vi "StartCapture.vi"(0 "object in":refnum<class "Hamamatsu.lvclass">, 5 "error in (no error)":errorcluster) -> (14 "object out":refnum<class "Hamamatsu.lvclass">, 19 "error out":errorcluster)   [LabVIEW 2019, in "Hamamatsu.lvclass"]
uses:
  Hamamatsu.lvclass
  Hamamatsu.lvclass/Hamamatsu.ctl
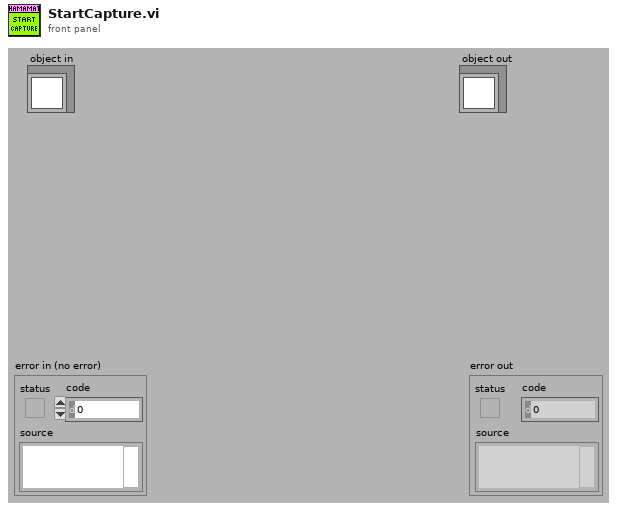
[diagram p1: front panel]
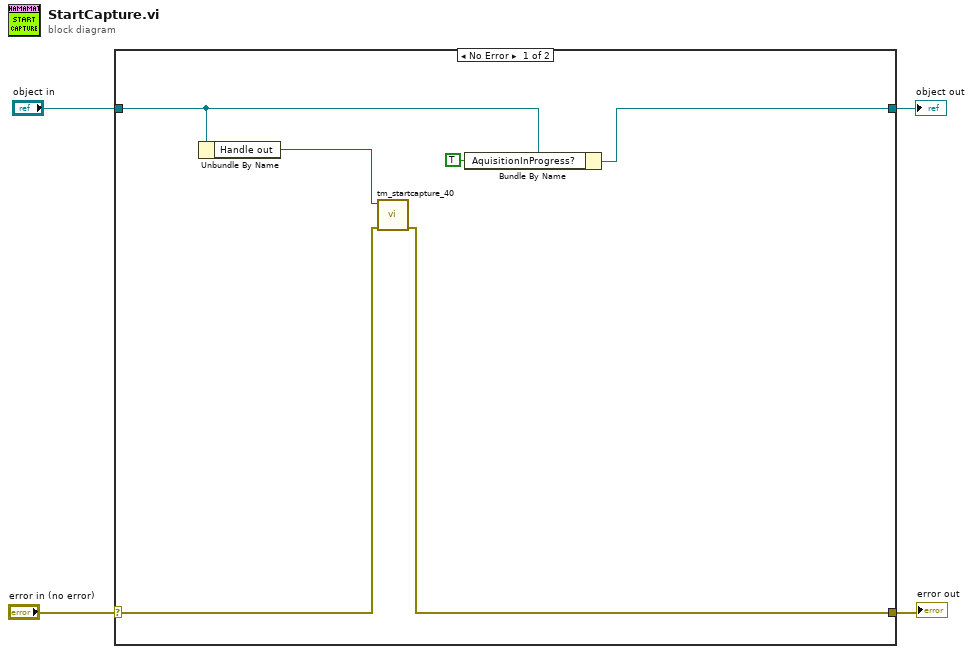
[diagram p0: block diagram]
diagram:
  n1 = case shown="No Error" "error in (no error)" {
    selector: "error in (no error)" -> [w9 w12]
    tunnel: [w8 w12] -> w3
    tunnel: [w7 w11] -> w1
    tunnel: "object in" -> [w6 w11]
    frame No Error {
      n2 = Unbundle By Name(w6) -> ("Handle out"=w10:u32)
      n3 = call <userlib>:"tm_startcapture_40.vi"("error in (no error)"=w9, "Handle in"=w10) -> ("error out"=w8:errorcluster)  [unwired: 8 in, 1 out]
      n4 = Bundle By Name(cluster=w6, "AquisitionInProgress?"=TRUE ("CameraConnected?")) -> (w7:refnum<class "Hamamatsu.lvclass">)
    }
    frame Error {
    }
  }
  "error out" <- w3
  "object out" <- w1
